vi "CSM - Append Continious State.vi"(6 "Loop State(s) and Arguments":string, 9 "Continous Arguments (\"\")":string, 10 "Continous State":string, 11 "Remaining States":string) -> (3 "States Out":string)   [LabVIEW 2014, in "CSM Loop Support.lvlib"]
uses:
  CSM Loop Support.lvlib
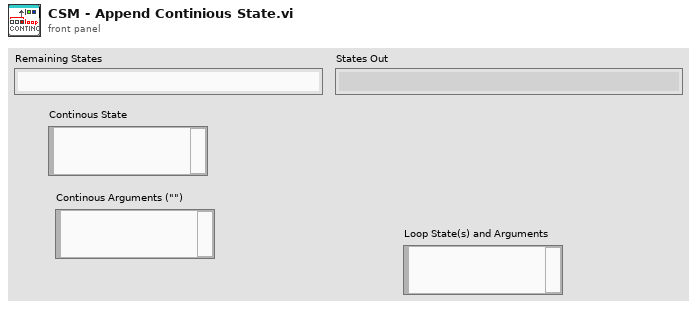
[diagram p1: front panel]
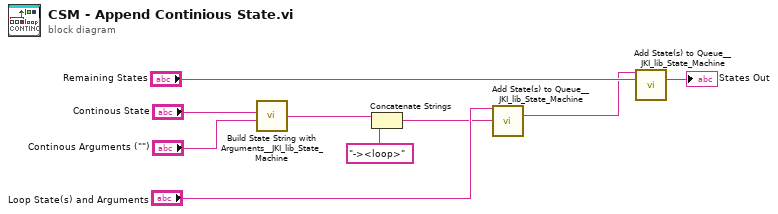
[diagram p0: block diagram]
diagram:
  n1 = call <vilib>:"Build State String with Arguments__JKI_lib_State_Machine.vi"("Arguments (\"\")"="Continous Arguments (\"\")", "State"="Continous State") -> ("State with Arguments"=w5:string)  [unwired: 4 in]
  n2 = Concatenate Strings(w5, "-><loop>" ("string")) -> (w2:string)
  n3 = call <vilib>:"Add State(s) to Queue__JKI_lib_State_Machine.vi"("State(s) in Front (\"\")"="Loop State(s) and Arguments", "State(s) in (\"\")"=w2) -> ("States Out"=w3:string)  [unwired: 13 in]
  n4 = call <vilib>:"Add State(s) to Queue__JKI_lib_State_Machine.vi"("State(s) in Front (\"\")"=w3, "State(s) in (\"\")"="Remaining States") -> ("States Out"=→"States Out":string)  [unwired: 13 in]
